vi "ObtainItemsUsedInApp.vi"() -> ()   [LabVIEW 2016]
uses:
  <vilib>/Utility/traverseref.llb/TRef TravTarget.ctl
  <vilib>/Utility/traverseref.llb/VI Scripting - Traverse.lvlib
panel:
  out "CtrlReferences":refnum<vi>[](array[refnum])
  out "SubVIRefs":refnum<vi>[](array[refnum])
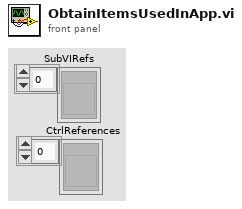
[diagram p1: front panel]
types:
  T1 = typedef "TRef TravTarget.ctl" = enum16{"FP", "BD", "Other"}
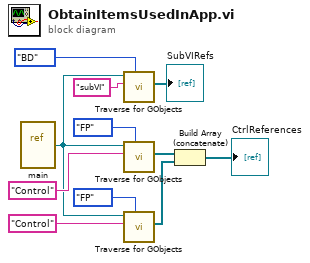
[diagram p0: block diagram]
diagram:
  n1 = vi-ref "main.vi"() -> (w4:refnum<vi>)
  n2 = call <vilib>:"Traverse for GObjects.vi"("Traverse Target"=TRef_TravTarget."BD", "Class Name"="subVI", "VI Refnum"=w4) -> ("References"=→"SubVIRefs":refnum<vi>[])  [unwired: 5 in, 3 out]
  n3 = call <vilib>:"Traverse for GObjects.vi"("Traverse Target"=TRef_TravTarget."FP", "Class Name"="Control", "VI Refnum"=w4) -> ("References"=w3:refnum<vi>[])  [unwired: 5 in, 3 out]
  n4 = call <vilib>:"Traverse for GObjects.vi"("Traverse Target"=TRef_TravTarget."FP", "Class Name"="Control", "VI Refnum"=w4) -> ("References"=w2:refnum<vi>[])  [unwired: 5 in, 3 out]
  n5 = Build Array (concatenate)(w3, w2) -> (→"CtrlReferences":refnum<vi>[])
